vi "FTW-Connector-LaunchActor.vi"(0 "FTW Actor Connector Type":refnum<class "FTW-ActorConnector.lvclass">, 5 "Configuration":T1, 7 "Actor VI Filepath":path, 11 "error in":errorcluster) -> (4 "FTW Actor Connector":refnum<class "FTW-ActorConnector.lvclass">, 15 "error out":errorcluster)   [LabVIEW 2012, in "FTW-Actor.lvlib" / "FTW-ActorConnector.lvclass"]
uses:
  FTW-ActorConnector.lvclass
  Utility/FTW-Actor-Configuration.ctl
  <instcachedir>/0/FTW-JSON-ToLabVIEW_0E3E72F634BF4A9AB33E22111E055A26.lvgen/FTW-JSON-ToLabVIEW_0E3E72F634BF4A9AB33E22111E055A26_002.vi
  Core/JSON/FTW-JSON-RegexParse.vi
  Core/Regex/FTW-Regex.vi
  Core/JSON/FTW-JSON-RegexHeader.vi
  Core/Error/FTW-ERR-ThrowError.vi
  Core/Error/FTW-ERR-ThrowGenericError.vi
  Core/Container/FTW-Container-Construct.vi
  Core/Container/FTW-Container-Load-JSON.vi
  Core/Container/FTW-Container-Destroy.vi
  FTW-Actor.lvlib
panel:
  # "Inputs"
  # "Outputs"
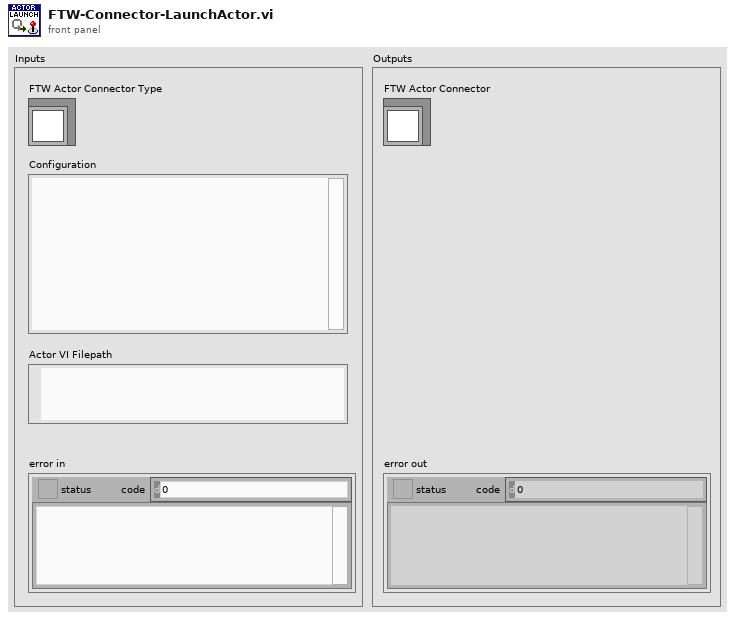
[diagram p1: front panel]
types:
  T1 = typedef "FTW-Actor.lvlib/FTW-Actor-Configuration.ctl" = string
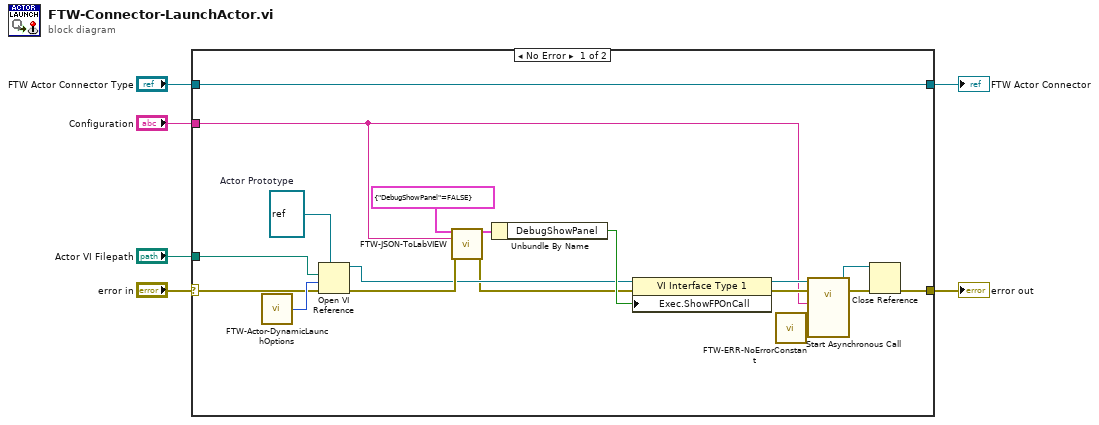
[diagram p0: block diagram]
diagram:
  n1 = case shown="No Error" "error in" {
    selector: "error in" -> [w20 w26]
    tunnel: [w22 w26] -> w6
    tunnel: "Configuration" -> [w10 _]
    tunnel: [w21 w25] -> w3
    tunnel: "FTW Actor Connector Type" -> [w21 w25]
    tunnel: "Actor VI Filepath" -> [w19 _]
    frame No Error {
      w24 = refnum<vi> refnum  # Actor Prototype
      n2 = call "FTW-Actor-DynamicLaunchOptions.vi"() -> ("Open VI Ref Options"=w23:i32)
      n3 = Open VI Reference(type specifier VI Refnum (for type only)=w24, vi path=w19, options=w23, error in (no error)=w20) -> (vi reference=w8:refnum<vi>, error out=w11:errorcluster)  [unwired: 2 in]
      n4 = call-generic "FTW-JSON-ToLabVIEW.vi"("Type and Defaults"=cluster{"DebugShowPanel":bool} {"DebugShowPanel"=FALSE}, "JSON String"=w10, "error in"=w11) -> ("Populated Values"=w12:cluster{"DebugShowPanel":bool}, "error out"=w7:errorcluster)  [unwired: 11 in]
      n5 = Unbundle By Name(w12) -> ("DebugShowPanel"=w9:bool)
      n6 = property class="VI Interface Type 1"(reference=w8, error in=w7, "Exec.ShowFPOnCall"=w9) -> (reference out=w15:refnum<vi>, error out=w14:errorcluster)
      n7 = call "FTW-ERR-NoErrorConstant.vi"() -> ("no error"=w18:errorcluster)
      n8 = call-by-ref "Start Asynchronous Call"(reference=w15, error in=w14, "Configuration"=w10, "ErrorIn"=w18) -> (reference out=w17:refnum<vi>, error out=w16:errorcluster)  [unwired: 13 in, 1 out]
      n9 = Close Reference(reference=w17, error in (no error)=w16) -> (error out=w22:errorcluster)
    }
    frame Error {
    }
  }
  "error out" <- w6
  "FTW Actor Connector" <- w3
